vi "6.写入文本文件不覆盖.vi"() -> ()   [LabVIEW 2018]
panel:
  out "文本":string
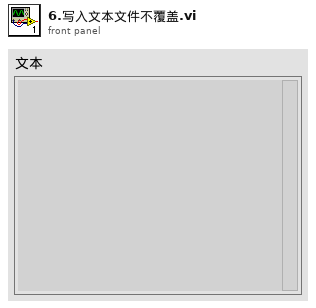
[diagram p1: front panel]
types:
  T1 = enum16{"open", "replace", "create", "open or create", "replace or create", "replace or create with confirmation"}
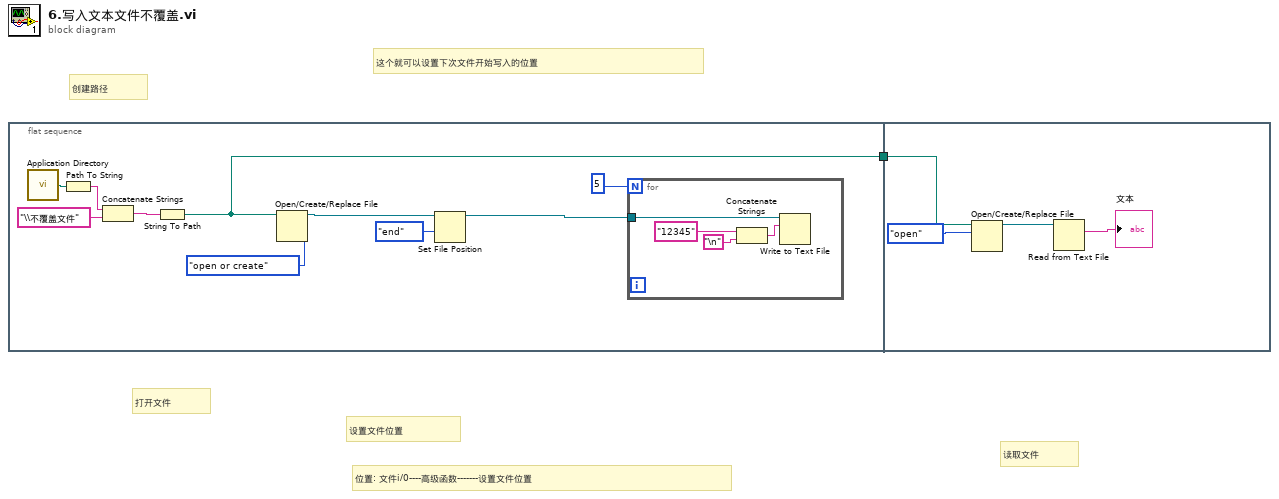
[diagram p0: block diagram]
diagram:
  # "读取文件"
  # "打开文件"
  # "这个就可以设置下次文件开始写入的位置"
  # "位置: 文件i/0----高级函数-------设置文件位置"
  # "设置文件位置"
  # "创建路径"
  n1 = flat-sequence {
    tunnel: [w2] -> w1
    tunnel: w1 -> [w18]
    frame #0 {
      n2 = call <vilib>:"Application Directory.vi"() -> ("Application Directory"=w11:path)
      n3 = Path To String(path=w11) -> (string=w10:string)
      n4 = Concatenate Strings(w10, "\\不覆盖文件") -> (w8:string)
      n5 = String To Path(string=w8) -> (path=w2:path)
      n6 = Open/Create/Replace File(file path (use dialog)=w2, operation (0:open)=T1."open or create" ("操作(0:open)")) -> (refnum out=w6:refnum<file>)  [unwired: 4 in, 2 out]
      n7 = Set File Position(refnum=w6, from (0:start)=enum16{"start", "end", "current"}."end" ("自（0:起始）")) -> (refnum out=w3:refnum<file>)  [unwired: 2 in, 1 out]
      n8 = for {
        N: 5 -> [_]
        tunnel: w3 -> [w15]
        n9 = Concatenate Strings("12345" ("文本"), "\n") -> (w12:string)
        n10 = Write to Text File(file (use dialog)=w15, text=w12) -> ()  [unwired: 2 in, 3 out]
      }
    }
    frame #1 {
      n11 = Open/Create/Replace File(file path (use dialog)=w18, operation (0:open)=T1."open" ("操作(0:open)")) -> (refnum out=w19:refnum<file>)  [unwired: 4 in, 2 out]
      n12 = Read from Text File(file (use dialog)=w19) -> (text=→"文本":string)  [unwired: 3 in, 3 out]
    }
  }
